vi "MegaAnalysis5.vi"() -> ()   [LabVIEW 2016] (continued)
                        tunnel: w4729 -> [w4829 w4834 w4839 w4845]
                        frame 0, Default {
                          n1882 = call "readbinary.vi"(7:w4829, "base path"=w4831, "file index"=w4832, "data column"="timi") -> ("data"=w4830:ext[])  [unwired: 7 out]
                        }
                        frame 1 {
                          n1883 = call "readbinary.vi"(7:w4834, "base path"=w4836, "file index"=w4837, "data column"="bcli") -> ("data"=w4835:ext[])  [unwired: 7 out]
                        }
                        frame 2 {
                          n1884 = call "readbinary.vi"(7:w4839, "base path"=w4842, "file index"=w4843, "data column"="bcli") -> ("data"=w4841:ext[])  [unwired: 7 out]
                          n1885 = Reciprocal(x=w4841) -> (1/x=w4840:ext[])
                        }
                        frame 3 {
                          n1886 = call "readbinary.vi"(7:w4845, "base path"=w4847, "file index"=w4848, "data column"="dati") -> ("data"=w4846:ext[])  [unwired: 7 out]
                        }
                      }
                      n1887 = case shown="2" w4736 {
                        tunnel: w4730 -> [w4811 w4816 w4822 w4827]
                        tunnel: w4732 -> [w4810 w4815 w4821 w4826]
                        tunnel: [w4809 w4814 w4819 w4825] -> w4727
                        tunnel: w4729 -> [w4808 w4813 w4818 w4824]
                        frame 0, Default {
                          n1888 = call "readbinary.vi"(7:w4808, "base path"=w4810, "file index"=w4811, "data column"="timi") -> ("data"=w4809:ext[])  [unwired: 7 out]
                        }
                        frame 1 {
                          n1889 = call "readbinary.vi"(7:w4813, "base path"=w4815, "file index"=w4816, "data column"="bcli") -> ("data"=w4814:ext[])  [unwired: 7 out]
                        }
                        frame 2 {
                          n1890 = call "readbinary.vi"(7:w4818, "base path"=w4821, "file index"=w4822, "data column"="bcli") -> ("data"=w4820:ext[])  [unwired: 7 out]
                          n1891 = Reciprocal(x=w4820) -> (1/x=w4819:ext[])
                        }
                        frame 3 {
                          n1892 = call "readbinary.vi"(7:w4824, "base path"=w4826, "file index"=w4827, "data column"="dati") -> ("data"=w4825:ext[])  [unwired: 7 out]
                        }
                      }
                      n1893 = Array Max & Min(array=w4727) -> (min value=w4726:ext)  [unwired: 3 out]
                      n1894 = case shown="0, Default" w4735 {
                        tunnel: w4734 -> [w4789 w4806]
                        tunnel: w4727 -> [w4786 w4807]
                        tunnel: w4733 -> [w4759 _]
                        tunnel: w4730 -> [w4770 w4802]
                        tunnel: w4732 -> [w4772 w4801]
                        tunnel: w4731 -> [w4768 _]
                        tunnel: w4728 -> [w4757 w4794]
                        tunnel: w4726 -> [w4749 _]
                        tunnel: w4725 -> [w4742 _]
                        frame 0, Default {
                          w4762 = 0
                          n1895 = Array Size(array=w4786) -> (size(s)=w4779:i32)
                          n1896 = Index Array(array=w4786, index=0) -> (element=w4784:ext)
                          n1897 = Decrement(x=w4779) -> (x-1=w4787:i32)
                          n1898 = Index Array(array=w4786, index=w4787) -> (element=w4783:ext)
                          n1899 = Subtract(x=w4784, y=w4783) -> (x-y=w4782:ext)
                          n1900 = Scale By Power Of 2(n=w4759, x=w4779) -> (x*2^n=w4766:i32)
                          n1901 = call-poly <vilib>:"Scaled Time Domain Window.vi"("window"="FT window", "X"=w4789) -> ("Windowed X"=w4750:dbl[])  [unwired: 1 in, 8 out]
                          n1902 = Scale By Power Of 2(n=w4759, x=1) -> (x*2^n=w4758:i32)
                          n1903 = Reciprocal(x=w4782) -> (1/x=w4780:ext)
                          n1904 = Subtract(x=w4766, y=w4779) -> (x-y=w4777:i32)
                          n1905 = Absolute Value(x=w4780) -> (abs(x)=w4781:ext)
                          n1906 = Array Size(array=w4750) -> (size(s)=w4755:i32)
                          n1907 = Divide(x=w4781, y=w4758) -> (x/y=w4775:ext)
                          n1908 = for {
                            N: w4777 -> [_]
                            tunnel: [0] -> w4778 mode=indexing
                          }
                          n1909 = Build Array (concatenate)(w4750, w4778) -> (w4756:dbl[])
                          n1910 = Divide(x=w4755, y=2) -> (x/y=w4753:dbl)
                          n1911 = call-poly <vilib>:"FFT.vi"("X"=w4756) -> ("FFT {X}"=w4752:cdb[])  [unwired: 2 in, 8 out]
                          n1912 = Divide(x=w4752, y=w4753) -> (x/y=w4751:cdb[])
                          n1913 = Complex To Polar(r * e^(i*theta)=w4751) -> (r=w4765:dbl[], theta=w4764:dbl[])
                          n1914 = for {
                            N: w4766 -> [w4790]
                            tunnel: [0] -> _ mode=indexing
                            tunnel: [w4791] -> w4776 mode=indexing
                            tunnel: [w4790] -> _ mode=indexing
                            i -> [w4791]
                          }
                          n1915 = Multiply(x=w4775, y=w4776) -> (x*y=w4763:ext[])
                          n1916 = Scale By Power Of 2(n=w4768, x=1) -> (x*2^n=w4767:i32)
                          n1917 = Divide(x=w4766, y=w4767) -> (x/y=w4761:dbl)
                          n1918 = Array Subset(array=w4765, index=w4762, length=w4761) -> (w4740:dbl[])
                          n1919 = Array Subset(array=w4764, index=w4762, length=w4761) -> (w4745:dbl[])
                          n1920 = Array Subset(array=w4763, index=w4762, length=w4761) -> (w4748:ext[])
                          n1921 = Multiply(x=w4748, y=w4749) -> (x*y=w4747:ext[])
                          n1922 = Multiply(x=w4747, y=6.283185307179586) -> (x*y=w4744:ext[])
                          n1923 = Multiply(x=w4744, y=w4742) -> (x*y=w4743:ext[])
                          n1924 = Subtract(x=w4745, y=w4743) -> (x-y=w4741:ext[])
                          n1925 = Polar To Complex(1:w4741, 2:w4740) -> (0:w4739:cxt[])
                          n1926 = call "writebinary.vi"(7:w4757, "base path"=w4772, "file index"=w4770, "data column"="freq", "data"=w4748) -> ()  [unwired: 7 out]
                          n1927 = Complex To Polar(r * e^(i*theta)=w4739) -> (theta=w4738:ext[])  [unwired: 1 out]
                          n1928 = call "writebinary.vi"(7:w4757, "base path"=w4772, "file index"=w4770, "data column"="ampl", "data"=w4740) -> ()  [unwired: 7 out]
                          n1929 = call "writebinary.vi"(7:w4757, "base path"=w4772, "file index"=w4770, "data column"="phas", "data"=w4738) -> ()  [unwired: 7 out]
                        }
                        frame 1 {
                          n1930 = call "MaxEnt03.vi"("t"=w4807, "data"=w4806, "m"="Maximum Entropy M", "pad factor?"="Increase spectral density") -> ("f"=w4800:dbl[], "P"=w4799:dbl[])  [unwired: 3 out]
                          n1931 = Square Root(x=w4799) -> (sqrt(x)=w4798:dbl[])
                          n1932 = call "writebinary.vi"(7:w4794, "base path"=w4801, "file index"=w4802, "data column"="freq", "data"=w4800) -> ()  [unwired: 7 out]
                          n1933 = call "writebinary.vi"(7:w4794, "base path"=w4801, "file index"=w4802, "data column"="ampl", "data"=w4798) -> ()  [unwired: 7 out]
                          n1934 = call "writebinary.vi"(7:w4794, "base path"=w4801, "file index"=w4802, "data column"="phas", "data"=dbl[] [] ("Array 16")) -> ()  [unwired: 7 out]
                        }
                      }
                    }
                  }
                  frame #2 {
                    n1935 = case shown="True" "?" {
                      tunnel: "peak finder threshold" -> [_ w4859]
                      tunnel: "width" -> [_ w4858]
                      tunnel: w4852 -> [_ w4861]
                      tunnel: w4851 -> [_ w4860]
                      tunnel: w4850 -> [_ w4856]
                      frame False {
                      }
                      frame True {
                        n1936 = for {
                          tunnel: w4861 -> [_] mode=indexing
                          tunnel: w4860 -> [w4878]
                          tunnel: w4859 -> [w4880]
                          tunnel: w4858 -> [w4871]
                          tunnel: [w4866] -> w4857 mode=indexing
                          tunnel: w4856 -> [w4862]
                          i -> [w4879]
                          (unwired) 0
                          n1937 = call "readbinary.vi"(7:w4862, "base path"=w4878, "file index"=w4879, "data column"="freq") -> ("data"=w4870:ext[])  [unwired: 7 out]
                          n1938 = call "readbinary.vi"(7:w4862, "base path"=w4878, "file index"=w4879, "data column"="ampl") -> ("data"=w4881:ext[])  [unwired: 7 out]
                          n1939 = call "readbinary.vi"(7:w4862, "base path"=w4878, "file index"=w4879, "data column"="phas") -> ("data"=w4869:ext[])  [unwired: 7 out]
                          n1940 = Index Array(array=w4870) -> (element=w4873:ext)  [unwired: 1 in]
                          n1941 = Index Array(array=w4870, index=1) -> (element=w4874:ext)
                          n1942 = Subtract(x=w4874, y=w4873) -> (x-y=w4872:ext)
                          n1943 = Divide(x=w4872, y=w4871) -> (x/y=w4868:ext)
                          n1944 = call-poly <vilib>:"Waveform Peak Detection.vi"("width"=w4868, "threshold"=w4880, "Signal In"=w4881) -> ("Amplitudes"=w4864:dbl[], "Locations"=w4867:dbl[])  [unwired: 4 in, 3 out]
                          n1945 = for {
                            tunnel: w4870 -> [w4888]
                            tunnel: w4869 -> [w4887]
                            tunnel: w4867 -> [w4886] mode=indexing
                            tunnel: w4867 -> [w4885] mode=indexing
                            tunnel: [w4884] -> w4865 mode=indexing
                            tunnel: [w4883] -> w4863 mode=indexing
                            n1946 = Index Array(array=w4888, index=w4885) -> (element=w4884:ext)
                            n1947 = Index Array(array=w4887, index=w4886) -> (element=w4883:ext)
                          }
                          n1948 = Bundle(w4863, w4865, "Amplitudes"=w4864) -> (w4866:cluster{ext[], ext[], "Amplitudes":dbl[]})  [unwired: 1 out]
                        }
                        "peaks" <- w4857
                      }
                    }
                  }
                }
              }
            }
          }
          frame #2 {
            n1949 = Equal?(x=w4899, y=4) -> (x = y?=w4896:bool)
            n1950 = Equal?(x="?", y=1) -> (x = y?=w4897:bool)
            n1951 = Build Path(base path=w4891, name or relative path="files4") -> (appended path=w4893:path)
            n1952 = call-poly <vilib>:"Read From Spreadsheet File.vi"("file path (dialog if empty)"=w4893) -> ("first row"=w4892:string[])  [unwired: 3 in, 7 out]
            n1953 = And(x=w4897, y=w4896) -> (x .and. y?=w4902:bool)
            n1954 = case shown="True" w4902 {
              tunnel: "y axis" -> [_ w4912]
              tunnel: w4892 -> [_ w4914]
              tunnel: w4891 -> [_ w4913]
              tunnel: [w4906 w4911] -> w4890
              tunnel: w4889 -> [_ w4910]
              frame False {
                w4908 = dbl[] [] ("Array 15")
                n1955 = Bundle("Array 15"=w4908, "Array 15"=w4908) -> (w4907:cluster{"Array 15":dbl[], "Array 15":dbl[]})  [unwired: 1 out]
                n1956 = Build Array(w4907) -> (w4906:cluster{"Array 15":dbl[], "Array 15":dbl[]}[])
              }
              frame True {
                n1957 = for {
                  tunnel: w4914 -> [_] mode=indexing
                  tunnel: w4913 -> [w4919]
                  tunnel: w4912 -> [w4921]
                  tunnel: [w4916] -> w4911 mode=indexing
                  tunnel: w4910 -> [w4915]
                  i -> [w4920]
                  n1958 = call "readbinary.vi"(7:w4915, "base path"=w4919, "file index"=w4920, "data column"="freq") -> ("data"=w4918:ext[])  [unwired: 7 out]
                  n1959 = case shown="2" w4921 {
                    tunnel: w4920 -> [w4926 w4932 w4937]
                    tunnel: w4919 -> [w4925 w4931 w4936]
                    tunnel: [w4924 w4929 w4935] -> w4917
                    tunnel: w4915 -> [w4923 w4928 w4934]
                    frame 0, Default {
                      n1960 = call "readbinary.vi"(7:w4923, "base path"=w4925, "file index"=w4926, "data column"="ampl") -> ("data"=w4924:ext[])  [unwired: 7 out]
                    }
                    frame 1 {
                      n1961 = call "readbinary.vi"(7:w4928, "base path"=w4931, "file index"=w4932, "data column"="ampl") -> ("data"=w4930:ext[])  [unwired: 7 out]
                      n1962 = Multiply(x=w4930, y=w4930) -> (x*y=w4929:ext[])
                    }
                    frame 2 {
                      n1963 = call "readbinary.vi"(7:w4934, "base path"=w4936, "file index"=w4937, "data column"="phas") -> ("data"=w4935:ext[])  [unwired: 7 out]
                    }
                  }
                  n1964 = Bundle("data"=w4918, "data"=w4917) -> (w4916:cluster{"data":ext[], "data":ext[]})  [unwired: 1 out]
                }
                n1965 = global write "status.vi" "String"("plotting transform") -> ()
              }
            }
            "?" <- w4890
            n1966 = while {
              stop <- w4904 stop-if-true
              n1967 = Not(x="?") -> (.not. x?=w4904:bool)
              n1968 = Wait (ms)(milliseconds to wait=1000) -> ()  [unwired: 1 out]
            }
          }
          frame #3 {
            w4941 = FALSE  # Set axes names
            n1969 = Build Path(base path=w4948, name or relative path="files4") -> (appended path=w4955:path)
            n1970 = Build Path(base path=w4948, name or relative path="paths4") -> (appended path=w4953:path)
            n1971 = call-poly <vilib>:"Read From Spreadsheet File.vi"("file path (dialog if empty)"=w4953) -> ("first row"=w4952:string[])  [unwired: 3 in, 7 out]
            n1972 = Build Array("freq", "ampl", "phas") -> (w4950:string[])
            n1973 = call-poly <vilib>:"Read From Spreadsheet File.vi"("file path (dialog if empty)"=w4955) -> ("first row"=w4944:string[])  [unwired: 3 in, 7 out]
            "files 2" <- w4944
            n1974 = case shown="0, Default" "label" {
              tunnel: w4944 -> [w4962 _ _]
              tunnel: [w4962 w4965 w4970] -> w4939
              frame 0, Default {
              }
              frame 1 {
                n1975 = property on="angle theta (cos theta renorm.)" class="Arr (strict)"() -> ("Value"=w4966:ext[])  [unwired: 2 in, 2 out]
                n1976 = Number To Fractional String(number=w4966, width (-)=10, precision (6)=3) -> (F-format string=w4965:string[])  [unwired: 1 out]
              }
              frame 2 {
                n1977 = property on="variable (T)" class="Arr (strict)"() -> ("Value"=w4969:dbl[])  [unwired: 2 in, 2 out]
                n1978 = Number To Fractional String(number=w4969, width (-)=10, precision (6)=3) -> (F-format string=w4970:string[])  [unwired: 1 out]
              }
            }
            n1979 = String To Path(string=w4952) -> (path=w4951:path[])
            n1980 = case shown="True" "?" {
              tunnel: w4944 -> [_ w4981]
              tunnel: w4951 -> [_ w4980]
              tunnel: w4950 -> [_ w4979]
              tunnel: w4948 -> [_ w4973]
              tunnel: "file format" -> [_ w4978]
              tunnel: "append name" -> [_ w4977]
              tunnel: w4947 -> [_ w4976]
              tunnel: w4946 -> [w4971 w4975]
              tunnel: [w4971 w4974] -> w4945
              frame False {
              }
              frame True {
                n1981 = for {
                  tunnel: w4981 -> [w4998] mode=indexing
                  tunnel: w4980 -> [w4996] mode=indexing
                  tunnel: w4977 -> [w4997]
                  tunnel: w4979 -> [w4994]
                  tunnel: w4973 -> [w4992]
                  tunnel: w4978 -> [w4989]
                  tunnel: w4976 -> [w4988]
                  shift-right: [w4984] -> w4974
                  shift-left: w4975 -> [w4986]
                  tunnel: w4973 -> [w4982]
                  i -> [w4993]
                  n1982 = call "filecount.vi"("Path"=w4982) -> ("file count string"=w4983:string)  [unwired: 10 in]
                  n1983 = Concatenate Strings("mega", w4983, w4998, w4997) -> (w4995:string)
                  n1984 = Build Path(base path=w4996, name or relative path=w4995) -> (appended path=w4985:path)
                  n1985 = Build Array (concatenate)(w4985, w4986) -> (w4984:path[])
                  n1986 = for {
                    tunnel: w4994 -> [w5010] mode=indexing
                    tunnel: w4993 -> [w5013]
                    tunnel: w4992 -> [w5012]
                    tunnel: [w5011] -> w4990 mode=indexing
                    tunnel: w4988 -> [w5009]
                    n1987 = call "readbinary.vi"(7:w5009, "base path"=w5012, "file index"=w5013, "data column"=w5010) -> ("data"=w5011:ext[])  [unwired: 7 out]
                  }
                  n1988 = stacked-sequence {
                    tunnel: "frequency\tamplitude\tphase\n" -> [_ w5004 _]
                    tunnel: w4985 -> [w4999 w5003 w5007]
                    tunnel: w4990 -> [_ _ w5008]
                    tunnel: w4989 -> [_ _ w5006]
                    frame #0 {
                      n1989 = call <vilib>:"Check if File or Folder Exists.vi"("path"=w4999) -> ("file or folder exists?"=w5000:bool)  [unwired: 1 in, 9 out]
                      n1990 = case shown="True" w5000 {
                        selector: w5000 -> [_ w5002]
                        tunnel: w4999 -> [_ w5001]
                        frame False {
                        }
                        frame True {
                          n1991 = Delete(path (use dialog)=w5001, entire hierarchy (F)=w5002) -> ()  [unwired: 1 in, 5 out]
                        }
                      }
                    }
                    frame #1 {
                      n1992 = Write to Text File(file (use dialog)=w5003, text=w5004) -> ()  [unwired: 1 in, 4 out]
                    }
                    frame #2 {
                      w5005 = TRUE
                      n1993 = call "Write To Spreadsheet File2.vi"("transpose? (no:F)"=w5005, "format (%d)"=w5006, "append to file? (new file:F)"=w5005, "2D data"=w5008, "file path (dialog if empty)"=w5007) -> ()  [unwired: 3 in, 1 out]
                    }
                  }
                }
                n1994 = global write "status.vi" "String"("saving transform") -> ()
              }
            }
            n1995 = control-ref of="?"() -> (w4940:refnum<vi>)
            n1996 = call "Neilsetplot.vi"("Set axes names"=w4941, "max # rows (-1:all)"=-1, "Plot names"=w4939, "XYGraph Refnum"=w4940) -> ()  [unwired: 6 in, 2 out]
          }
        }
      }
      frame #8 {
        # "analysis frame"
        n1997 = Build Path(base path=w5014, name or relative path="files3") -> (appended path=w5026:path)
        n1998 = Build Path(base path=w5014, name or relative path="files4") -> (appended path=w5034:path)
        n1999 = Equal?(x="?", y=1) -> (x = y?=w5029:bool)
        n2000 = call-poly <vilib>:"Read From Spreadsheet File.vi"("file path (dialog if empty)"=w5026) -> ("first row"=w5024:string[])  [unwired: 3 in, 7 out]
        n2001 = Equal?(x=w5030, y=5) -> (x = y?=w5028:bool)
        n2002 = call-poly <vilib>:"Read From Spreadsheet File.vi"("file path (dialog if empty)"=w5034) -> ("first row"=w5017:string[])  [unwired: 3 in, 7 out]
        n2003 = for {
          tunnel: w5017 -> [_] mode=indexing
          tunnel: [w5038] -> w5020 mode=indexing
          i -> [w5038]
        }
        n2004 = Number To Decimal String(number=w5020, width (-)=3) -> (decimal integer string=w5018:string[])
        n2005 = And(x=w5029, y=w5028) -> (x .and. y?=w5027:bool)
        n2006 = Build Array(w5018, w5017) -> (w5016:string[][])
        n2007 = Transpose 2D Array(2D array=w5016) -> (transposed array=→"file list":string[][])
        n2008 = stacked-sequence {
          tunnel: "?" -> [_ w5046 _ _]
          tunnel: w5036 -> [_ w5045 _ _]
          tunnel: w5014 -> [_ w5044 w5188 w5257]
          tunnel: w5017 -> [_ w5043 _ _]
          tunnel: w5027 -> [_ _ w5189 _]
          tunnel: w5024 -> [_ w5042 _ _]
          tunnel: w5023 -> [_ w5041 _ _]
          tunnel: w5022 -> [_ _ _ w5254]
          tunnel: [_ _ _ w5253] -> w5021
          frame #0 {
            n2009 = case shown="True" "set B angle as the variable?" {
              frame False {
              }
              frame True {
                n2010 = property on="angle theta (cos theta renorm.)" class="Arr (strict)"() -> ("Value"=w5040:ext[])  [unwired: 2 in, 2 out]
                n2011 = property on="variable (T)" class="Arr (strict)"("Val(Sgnl)"=w5040) -> ()  [unwired: 2 in, 2 out]
              }
            }
          }
          frame #1 {
            n2012 = case shown="True" w5046 {
              tunnel: w5044 -> [w5047 w5068]
              tunnel: w5045 -> [_ w5067]
              tunnel: w5043 -> [_ w5066]
              tunnel: w5042 -> [_ w5065]
              tunnel: w5041 -> [_ w5064]
              frame False {
                n2013 = Build Path(base path=w5047, name or relative path="afits") -> (appended path=w5052:path)
                n2014 = call <vilib>:"Check if File or Folder Exists.vi"("path"=w5052) -> ("file or folder exists?"=w5053:bool)  [unwired: 1 in, 9 out]
                n2015 = Build Path(base path=w5047, name or relative path="table") -> (appended path=w5055:path)
                n2016 = case shown="False" w5053 {
                  tunnel: w5052 -> [w5060 _]
                  frame False {
                    n2017 = call-poly <vilib>:"Write To Spreadsheet File.vi"("1D data"=string[] [] ("Array 20"), "file path (dialog if empty)"=w5060) -> ()  [unwired: 4 in, 3 out]
                  }
                  frame True {
                  }
                }
                n2018 = call <vilib>:"Check if File or Folder Exists.vi"("path"=w5055) -> ("file or folder exists?"=w5056:bool)  [unwired: 1 in, 9 out]
                n2019 = case shown="False" w5056 {
                  tunnel: w5055 -> [w5062 _]
                  frame False {
                    n2020 = call-poly <vilib>:"Write To Spreadsheet File.vi"("1D data"=string[] [] ("Array 18"), "file path (dialog if empty)"=w5062) -> ()  [unwired: 4 in, 3 out]
                  }
                  frame True {
                  }
                }
                n2021 = Build Path(base path=w5047, name or relative path="tfits") -> (appended path=w5049:path)
                n2022 = call <vilib>:"Check if File or Folder Exists.vi"("path"=w5049) -> ("file or folder exists?"=w5050:bool)  [unwired: 1 in, 9 out]
                n2023 = case shown="False" w5050 {
                  tunnel: w5049 -> [w5058 _]
                  frame False {
                    n2024 = call-poly <vilib>:"Write To Spreadsheet File.vi"("1D data"=string[] [] ("Array 21"), "file path (dialog if empty)"=w5058) -> ()  [unwired: 4 in, 3 out]
                  }
                  frame True {
                  }
                }
              }
              frame True {
                n2025 = stacked-sequence {
                  seq-local: [w5083 _] -> [_ w5131]
                  seq-local: ["variable (T)" _] -> [_ w5130]
                  tunnel: w5068 -> [w5086 w5133]
                  tunnel: w5067 -> [w5093 _]
                  tunnel: w5066 -> [w5087 _]
                  tunnel: w5065 -> [_ w5134]
                  tunnel: w5064 -> [_ w5132]
                  frame #0 {
                    w5072 = FALSE  # Set axes names
                    (unwired) 3
                    n2026 = for {
                      tunnel: w5087 -> [_] mode=indexing
                      tunnel: w5093 -> [w5109]
                      tunnel: w5086 -> [w5107]
                      tunnel: "variable (T)" -> [w5113] mode=indexing
                      tunnel: "frequencies" -> [w5114]
                      tunnel: [w5112] -> w5090 mode=indexing
                      tunnel: [w5111] -> w5083 mode=indexing
                      tunnel: "amplitude" -> [w5106]
                      tunnel: "phase" -> [w5104]
                      i -> [w5108]
                      n2027 = call "readbinary.vi"(7:w5109, "base path"=w5107, "file index"=w5108, "data column"="ampl") -> ("data"=w5102:ext[])  [unwired: 7 out]
                      n2028 = call "readbinary.vi"(7:w5109, "base path"=w5107, "file index"=w5108, "data column"="freq") -> ("data"=w5116:ext[])  [unwired: 7 out]
                      n2029 = call "readbinary.vi"(7:w5109, "base path"=w5107, "file index"=w5108, "data column"="phas") -> ("data"=w5103:ext[])  [unwired: 7 out]
                      n2030 = case shown="0, Default" w5106 {
                        tunnel: [w5119 w5120 w5125] -> w5105
                        tunnel: w5104 -> [_ w5123 w5128]
                        tunnel: w5103 -> [_ w5124 w5129]
                        tunnel: w5102 -> [w5119 w5122 w5127]
                        frame 0, Default {
                        }
                        frame 1 {
                          n2031 = Add(x=w5124, y=w5123) -> (x+y=w5121:ext[])
                          n2032 = Polar To Re/Im(2:w5121, 3:w5122) -> (1:w5120:ext[])  [unwired: 1 out]
                        }
                        frame 2 {
                          n2033 = Add(x=w5129, y=w5128) -> (x+y=w5126:ext[])
                          n2034 = Polar To Re/Im(2:w5126, 3:w5127) -> (0:w5125:ext[])  [unwired: 1 out]
                        }
                      }
                      n2035 = call <vilib>:"Interpolate 1D.vi"("method"="interpolation method", "xi"=w5114, "X"=w5116, "Y"=w5105) -> ("yi"=w5111:dbl[])  [unwired: 2 in, 5 out]
                      n2036 = Build Array (concatenate)(w5113, w5111) -> (w5112:dbl[])
                    }
                    n2037 = Build Array (concatenate)(0, "frequencies") -> (w5091:dbl[])
                    n2038 = control-ref of="?"() -> (w5070:refnum<vi>)
                    n2039 = Number To Fractional String(number="frequencies", width (-)=10, precision (6)=3) -> (F-format string=w5078:string[])  [unwired: 1 out]
                    n2040 = Build Array (concatenate)(w5091, w5090) -> (w5089:dbl[][])
                    n2041 = for {
                      tunnel: w5078 -> [w5101] mode=indexing
                      tunnel: [w5098] -> w5077 mode=indexing
                      tunnel: [w5097] -> w5076 mode=indexing
                      n2042 = Concatenate Strings("data ", w5101) -> (w5098:string)
                      n2043 = Concatenate Strings("fit ", w5101) -> (w5097:string)
                    }
                    n2044 = Build Path(base path=w5086, name or relative path="table") -> (appended path=w5084:path)
                    n2045 = call-poly <vilib>:"Write To Spreadsheet File.vi"("format (%.3f)"="%.9f", "2D data"=w5089, "file path (dialog if empty)"=w5084) -> ()  [unwired: 3 in, 3 out]
                    n2046 = Interleave 1D Arrays(w5077, w5076) -> (w5069:string[])
                    n2047 = call "Neilsetplot.vi"("Set axes names"=w5072, "max # rows (-1:all)"=20, "Plot names"=w5069, "XYGraph Refnum"=w5070) -> ()  [unwired: 6 in, 2 out]
                    n2048 = for {
                      tunnel: w5069 -> [w5096] mode=indexing
                      tunnel: [w5095] -> w5075 mode=indexing
                      n2049 = Bundle(w5096) -> (w5095:cluster{string})  [unwired: 1 in]
                    }
                    "frequencies" <- w5075
                    n2050 = for {
                      tunnel: [w5094] -> _ mode=indexing
                      tunnel: w5069 -> [_] mode=indexing
                      i -> [w5094]
                    }
                  }
                  frame #1 {
                    n2051 = case shown="False" "?" {
                      tunnel: w5134 -> [_ w5165]
                      tunnel: w5133 -> [w5136 w5149]
                      tunnel: w5132 -> [_ w5164]
                      tunnel: w5131 -> [_ w5162]
                      tunnel: w5130 -> [_ w5160]
                      frame False {
                        n2052 = Build Path(base path=w5136, name or relative path="afits") -> (appended path=w5141:path)
                        n2053 = call <vilib>:"Check if File or Folder Exists.vi"("path"=w5141) -> ("file or folder exists?"=w5142:bool)  [unwired: 1 in, 9 out]
                        n2054 = case shown="False" w5142 {
                          tunnel: w5141 -> [w5146 _]
                          frame False {
                            n2055 = call-poly <vilib>:"Write To Spreadsheet File.vi"("1D data"=string[] [] ("Array 22"), "file path (dialog if empty)"=w5146) -> ()  [unwired: 4 in, 3 out]
                          }
                          frame True {
                          }
                        }
                        n2056 = Build Path(base path=w5136, name or relative path="tfits") -> (appended path=w5138:path)
                        n2057 = call <vilib>:"Check if File or Folder Exists.vi"("path"=w5138) -> ("file or folder exists?"=w5139:bool)  [unwired: 1 in, 9 out]
                        n2058 = case shown="False" w5139 {
                          tunnel: w5138 -> [w5144 _]
                          frame False {
                            n2059 = call-poly <vilib>:"Write To Spreadsheet File.vi"("1D data"=string[] [] ("Array 23"), "file path (dialog if empty)"=w5144) -> ()  [unwired: 4 in, 3 out]
                          }
                          frame True {
                          }
                        }
                      }
                      frame True {
                        n2060 = for {
                          tunnel: w5165 -> [_] mode=indexing
                          tunnel: w5149 -> [w5184]
                          tunnel: w5164 -> [w5183]
                          tunnel: [w5173] -> w5163 mode=indexing
                          i -> [w5185]
                          n2061 = call "readbinary.vi"(7:w5183, "base path"=w5184, "file index"=w5185, "data column"="bcli") -> ("data"=w5181:ext[])  [unwired: 7 out]
                          n2062 = Array Max & Min(array=w5181) -> (max value=w5180:ext, min value=w5179:ext)  [unwired: 2 out]
                          n2063 = Reciprocal(x=w5179) -> (1/x=w5177:ext)
                          n2064 = Reciprocal(x=w5180) -> (1/x=w5178:ext)
                          n2065 = Add(x=w5178, y=w5177) -> (x+y=w5176:ext)
                          n2066 = Divide(x=w5176, y=2) -> (x/y=w5174:ext)
                          n2067 = Reciprocal(x=w5174) -> (1/x=w5173:ext)
                        }
                        n2068 = Transpose 2D Array(2D array=w5162) -> (transposed array=w5161:dbl[][])
                        n2069 = call-poly <vilib>:"Mean.vi"("X"=w5163) -> ("mean"=w5159:dbl)  [unwired: 1 out]
                        n2070 = for {
                          tunnel: w5161 -> [w5171] mode=indexing
                          tunnel: w5160 -> [w5172]
                          tunnel: w5159 -> [w5170]
                          tunnel: "points" -> [w5169]
                          tunnel: [w5168] -> w5157 mode=indexing
                          tunnel: [w5167] -> w5153 mode=indexing
                          tunnel: [w5166] -> w5148 mode=indexing
                          n2071 = call "sinh.vi"("# points"=w5169, "B"=w5170, "Amp"=w5171, "T"=w5172) -> ("mass"=w5168:dbl, "Amp"=w5166:dbl[], "T"=w5167:dbl[])  [unwired: 5 out]
                        }
                        n2072 = Absolute Value(x=w5157) -> (abs(x)=→"mass":dbl[])
                        n2073 = Build Path(base path=w5149, name or relative path="tfits") -> (appended path=w5154:path)
                        n2074 = call-poly <vilib>:"Write To Spreadsheet File.vi"("format (%.3f)"="%.9f", "2D data"=w5153, "file path (dialog if empty)"=w5154) -> ()  [unwired: 3 in, 3 out]
                        n2075 = Build Path(base path=w5149, name or relative path="afits") -> (appended path=w5150:path)
                        n2076 = call-poly <vilib>:"Write To Spreadsheet File.vi"("format (%.3f)"="%.9f", "2D data"=w5148, "file path (dialog if empty)"=w5150) -> ()  [unwired: 3 in, 3 out]
                      }
                    }
                  }
                }
                n2077 = global write "status.vi" "String"("amplitude analysis") -> ()
              }
            }
          }
          frame #2 {
            n2078 = case shown="False" w5189 {
              tunnel: w5188 -> [_ w5198]
              tunnel: [w5191 w5199] -> w5187
              tunnel: [0 3000] -> w5186
              frame False {
                w5193 = dbl[] [] ("Array 19")
                n2079 = Bundle("Array 19"=w5193, "Array 19"=w5193) -> (w5192:cluster{"Array 19":dbl[], "Array 19":dbl[]})  [unwired: 1 out]
                n2080 = Build Array(w5192) -> (w5191:cluster{"Array 19":dbl[], "Array 19":dbl[]}[])
              }
              frame True {
                w5222 = 1
                n2081 = Build Path(base path=w5198, name or relative path="tfits") -> (appended path=w5211:path)
                n2082 = Build Path(base path=w5198, name or relative path="afits") -> (appended path=w5208:path)
                n2083 = call-poly <vilib>:"Read From Spreadsheet File.vi"("format (%.3f)"="%.9f", "file path (dialog if empty)"=w5211) -> ("all rows"=w5205:dbl[][])  [unwired: 2 in, 7 out]
                n2084 = call-poly <vilib>:"Read From Spreadsheet File.vi"("format (%.3f)"="%.9f", "file path (dialog if empty)"=w5208) -> ("all rows"=w5204:dbl[][])  [unwired: 2 in, 7 out]
                n2085 = Build Path(base path=w5198, name or relative path="table") -> (appended path=w5227:path)
                n2086 = call-poly <vilib>:"Read From Spreadsheet File.vi"("format (%.3f)"="%.9f", "file path (dialog if empty)"=w5227) -> ("all rows"=w5218:dbl[][])  [unwired: 2 in, 7 out]
                n2087 = Index Array(array=w5218, index (col)=0) -> (element=w5216:dbl[])  [unwired: 1 in]
                n2088 = for {
                  tunnel: w5205 -> [w5249] mode=indexing
                  tunnel: w5204 -> [w5248] mode=indexing
                  tunnel: [w5247] -> w5197 mode=indexing
                  n2089 = Bundle("all rows"=w5249, "all rows"=w5248) -> (w5247:cluster{"all rows":dbl[], "all rows":dbl[]})  [unwired: 1 out]
                }
                n2090 = Array Size(array=w5218) -> (size(s)=w5224:i32[])
                n2091 = Index Array(array=w5224, index=1) -> (element=w5223:i32)
                n2092 = Index Array(array=w5224, index=0) -> (element=w5214:i32)
                n2093 = Array Subset(array=w5216, index=1, length=w5214) -> (w5213:dbl[])
                n2094 = global write "status.vi" "String"("plotting") -> ()
                n2095 = Decrement(x=w5214) -> ()  [unwired: 1 out]
                n2096 = Decrement(x=w5223) -> (x-1=w5221:i32)
                n2097 = Array Subset(array=w5218, index (row)=w5222, length (row)=w5214, index (col)=w5222, length (col)=w5221) -> (w5220:dbl[][])
                n2098 = Transpose 2D Array(2D array=w5220) -> (transposed array=w5219:dbl[][])
                n2099 = for {
                  tunnel: w5219 -> [w5251] mode=indexing
                  tunnel: w5213 -> [w5252]
                  tunnel: [w5250] -> w5196 mode=indexing
                  n2100 = Bundle(w5252, w5251) -> (w5250:cluster{dbl[], dbl[]})  [unwired: 1 out]
                }
                n2101 = Array Size(array=w5196) -> (size(s)=w5202:i32)
                n2102 = Multiply(x=2, y=w5202) -> (x*y=w5200:i32)
                n2103 = for {
                  N: w5200 -> [_]
                  tunnel: w5197 -> [w5232]
                  tunnel: w5196 -> [w5233]
                  shift-right: [w5235] -> _
                  shift-left: 0 -> [w5230]
                  tunnel: [w5231] -> w5199 mode=indexing
                  i -> [w5229]
                  n2104 = case shown="0, Default" w5230 {
                    tunnel: w5229 -> [w5239 w5246]
                    tunnel: w5233 -> [w5238 _]
                    tunnel: [w5236 w5242] -> w5231
                    tunnel: w5232 -> [_ w5243]
                    frame 0, Default {
                      n2105 = Divide(x=w5239, y=2) -> (x/y=w5237:dbl)
                      n2106 = Index Array(array=w5238, index=w5237) -> (element=w5236:cluster{dbl[], dbl[]})
                    }
                    frame 1 {
                      n2107 = Decrement(x=w5246) -> (x-1=w5245:i32)
                      n2108 = Divide(x=w5245, y=2) -> (x/y=w5244:dbl)
                      n2109 = Index Array(array=w5243, index=w5244) -> (element=w5242:cluster{"all rows":dbl[], "all rows":dbl[]})
                    }
                  }
                  n2110 = Subtract(x=1, y=w5230) -> (x-y=w5235:i32)
                }
              }
            }
            "?" <- w5187
            n2111 = Wait (ms)(milliseconds to wait=w5186) -> ()  [unwired: 1 out]
          }
          frame #3 {
            n2112 = Build Path(base path=w5257, name or relative path="paths4") -> (appended path=w5258:path)
            n2113 = call-poly <vilib>:"Read From Spreadsheet File.vi"("file path (dialog if empty)"=w5258) -> ("first row"=w5256:string[])  [unwired: 3 in, 7 out]
            n2114 = String To Path(string=w5256) -> (path=w5255:path[])
            n2115 = case shown="True" "?" {
              tunnel: w5257 -> [_ w5273]
              tunnel: w5255 -> [_ w5275]
              tunnel: w5254 -> [w5261 w5265]
              tunnel: [w5261 w5263] -> w5253
              frame False {
              }
              frame True {
                n2116 = Index Array(array=w5275, index=0) -> (element=w5268:path)
                n2117 = call "filecount.vi"("Path"=w5273) -> ("file count string"=w5271:string)  [unwired: 10 out]
                n2118 = Build Path(base path=w5273, name or relative path="table") -> (appended path=w5277:path)
                n2119 = call-poly <vilib>:"Read From Spreadsheet File.vi"("format (%.3f)"="%.9f", "file path (dialog if empty)"=w5277) -> ("all rows"=w5267:dbl[][])  [unwired: 2 in, 7 out]
                n2120 = Concatenate Strings("mega", w5271, "append name") -> (w5269:string)
                n2121 = Build Path(base path=w5268, name or relative path=w5269) -> (appended path=w5264:path)
                n2122 = Build Array (concatenate)(w5264, w5265) -> (w5263:path[])
                n2123 = call "Write To Spreadsheet File2.vi"("format (%d)"="file format", "2D data"=w5267, "file path (dialog if empty)"=w5264) -> ()  [unwired: 5 in, 1 out]
                n2124 = global write "status.vi" "String"("saving analysis") -> ()
              }
            }
          }
        }
      }
      frame #9 {
        n2125 = stacked-sequence {
          seq-local: [w5280 _ _ _ _ _ _ _] -> [_ _ _ _ _ _ w5529 _]
          seq-local: [_ w5287 _ _ _ _ _ _] -> [_ _ _ _ _ _ w5528 _]
          seq-local: [_ _ w5380 _ _ _ _ _] -> [_ _ _ _ _ _ w5527 _]
          seq-local: [_ _ _ w5434 _ _ _ _] -> [_ _ _ _ _ _ w5526 _]
          seq-local: [_ _ _ _ w5486 _ _ _] -> [_ _ _ _ _ _ w5525 _]
          seq-local: [_ _ _ _ _ w5505 _ _] -> [_ _ _ _ _ _ w5524 _]
          seq-local: [_ _ _ _ _ _ w5522 _] -> [_ _ _ _ _ _ _ w5533]
          seq-local: [_ _ _ _ _ _ w5519 _] -> [_ _ _ _ _ _ _ w5532]
          tunnel: "?" -> [_ _ _ _ _ _ _ w5534]
          frame #0 {
            # "transform"
            # "interpolate"
            # "select"
            # "filter"
            # "import"
            # "pruge"
            n2126 = property class="Bool (strict)"() -> ("Value"=w5286:bool)  [unwired: 2 in, 2 out]
            n2127 = property class="Bool (strict)"() -> ("Value"=w5285:bool)  [unwired: 2 in, 2 out]
            n2128 = property class="Bool (strict)"() -> ("Value"=w5283:bool)  [unwired: 2 in, 2 out]
            n2129 = property class="Bool (strict)"() -> ("Value"=w5284:bool)  [unwired: 2 in, 2 out]
            n2130 = property class="Bool (strict)"() -> ("Value"=w5281:bool)  [unwired: 2 in, 2 out]
            n2131 = property class="Bool (strict)"() -> ("Value"=w5282:bool)  [unwired: 2 in, 2 out]
            n2132 = Bundle("Value"=w5286, "Value"=w5285, "Value"=w5284, "Value"=w5283, "Value"=w5282, "Value"=w5281) -> (w5280:T19)  [unwired: 1 out]
          }
          frame #1 {
            n2133 = stacked-sequence {
              seq-local: [w5292 _ _ _ _ _] -> [_ _ _ _ _ w5379]
              seq-local: [_ w5293 _ _ _ _] -> [_ _ _ _ _ w5378]
              seq-local: [_ _ w5345 _ _ _] -> [_ _ _ _ _ w5377]
              seq-local: [_ _ _ w5356 _ _] -> [_ _ _ _ _ w5376]
              seq-local: [_ _ _ _ w5371 _] -> [_ _ _ _ _ w5375]
              tunnel: [_ _ _ _ _ w5374] -> w5291
              frame #0 {
                n2134 = property on="files to be imported" class="Arr (strict)"() -> ("Value"=w5292:path[])  [unwired: 2 in, 2 out]
              }
              frame #1 {
                # "integration pretrigger option"
                n2135 = stacked-sequence {
                  tunnel: [w5301 _ _ _ _] -> w5298
                  tunnel: [_ w5307 _ _ _] -> w5297
                  tunnel: [_ _ w5315 _ _] -> w5296
                  tunnel: [_ _ _ w5324 _] -> w5295
                  tunnel: [_ _ _ _ w5334] -> w5294
                  frame #0 {
                    n2136 = property on="time interval  (for series)" class="DigNum (strict)"() -> ("Value"=w5304:dbl)  [unwired: 2 in, 2 out]
                    n2137 = property on="time column selection" class="Arr (strict)"() -> ("Value"=w5303:u16[])  [unwired: 2 in, 2 out]
                    n2138 = property on="time column rescale" class="Arr (strict)"() -> ("Value"=w5302:ext[])  [unwired: 2 in, 2 out]
                    n2139 = property on="option" class="Ring (strict)"() -> ("Value"=w5305:u16)  [unwired: 2 in, 2 out]
                    n2140 = Bundle("Value"=w5305, "Value"=w5304, "Value"=w5303, "Value"=w5302) -> (w5301:T20)  [unwired: 1 out]
                  }
                  frame #1 {
                    n2141 = property on="dB/dt column rescale" class="Arr (strict)"() -> ("Value"=w5308:ext[])  [unwired: 2 in, 2 out]
                    n2142 = property on="dB/dt column selection" class="Arr (strict)"() -> ("Value"=w5309:u16[])  [unwired: 2 in, 2 out]
                    n2143 = property on="option" class="Ring (strict)"() -> ("Value"=w5310:u16)  [unwired: 2 in, 2 out]
                    n2144 = property class="Bool (strict)"() -> ("Value"=w5306:bool)  [unwired: 2 in, 2 out]
                    n2145 = Bundle("Value"=w5310, "Value"=w5309, "Value"=w5308, "Value"=w5306) -> (w5307:T21)  [unwired: 1 out]
                  }
                  frame #2 {
                    n2146 = local read "B column selection"() -> (w5311:u16[])
                    n2147 = property on="B column offset" class="Arr (strict)"() -> ("Value"=w5319:ext[])  [unwired: 2 in, 2 out]
                    n2148 = property on="angle theta (cos theta renorm.)" class="Arr (strict)"() -> ("Value"=w5320:ext[])  [unwired: 2 in, 2 out]
                    n2149 = property on="B column rescale" class="Arr (strict)"() -> ("Value"=w5321:ext[])  [unwired: 2 in, 2 out]
                    n2150 = property on="pretrigger time for integration" class="DigNum (strict)"() -> ("Value"=w5322:dbl)  [unwired: 2 in, 2 out]
                    n2151 = property on="option" class="Ring (strict)"() -> ("Value"=w5323:u16)  [unwired: 2 in, 2 out]
                    n2152 = property class="Bool (strict)"() -> ("Value"=w5317:bool)  [unwired: 2 in, 2 out]
                    n2153 = property class="Bool (strict)"() -> ("Value"=w5318:bool)  [unwired: 2 in, 2 out]
                    n2154 = property class="Bool (strict)"() -> ("Value"=w5316:bool)  [unwired: 2 in, 2 out]
                    n2155 = property class="Bool (strict)"() -> ("Value"=w5314:bool)  [unwired: 2 in, 2 out]
                    n2156 = property class="DigNum (strict)"() -> ("Value"=w5313:u32)  [unwired: 2 in, 2 out]
                    n2157 = property class="DigNum (strict)"() -> ("Value"=w5312:dbl)  [unwired: 2 in, 2 out]
                    n2158 = Bundle("Value"=w5323, "Value"=w5322, "B column selection"=w5311, "Value"=w5321, "Value"=w5320, "Value"=w5319, "Value"=w5318, "Value"=w5317, "Value"=w5316, "Value"=w5314, "Value"=w5313, "Value"=w5312) -> (w5315:T22)  [unwired: 1 out]
                  }
                  frame #3 {
                    # "rotate array"
                    n2159 = property on="pretrigger time for integration" class="DigNum (strict)"() -> ("Value"=w5332:dbl)  [unwired: 2 in, 2 out]
                    n2160 = property on="data column rescale" class="Arr (strict)"() -> ("Value"=w5328:ext[])  [unwired: 2 in, 2 out]
                    n2161 = property class="Bool (strict)"() -> ("Value"=w5331:bool)  [unwired: 2 in, 2 out]
                    n2162 = property on="data column selection" class="Arr (strict)"() -> ("Value"=w5329:u16[])  [unwired: 2 in, 2 out]
                    n2163 = property on="option" class="Ring (strict)"() -> ("Value"=w5333:u16)  [unwired: 2 in, 2 out]
                    n2164 = property class="DigNum (strict)"() -> ("Value"=w5330:i64)  [unwired: 2 in, 2 out]
                    n2165 = property on="data column offset" class="Arr (strict)"() -> ("Value"=w5327:ext[])  [unwired: 2 in, 2 out]
                    n2166 = property class="Bool (strict)"() -> ("Value"=w5326:bool)  [unwired: 2 in, 2 out]
                    n2167 = property class="Bool (strict)"() -> ("Value"=w5325:bool)  [unwired: 2 in, 2 out]
                    n2168 = Bundle("Value"=w5333, "Value"=w5332, "Value"=w5331, "Value"=w5330, "Value"=w5329, "Value"=w5328, "Value"=w5327, "Value"=w5326, "Value"=w5325) -> (w5324:T23)  [unwired: 1 out]
                  }
                  frame #4 {
                    n2169 = property on="pretrigger time for integration" class="DigNum (strict)"() -> ("Value"=w5342:dbl)  [unwired: 2 in, 2 out]
                    n2170 = property on="option" class="Ring (strict)"() -> ("Value"=w5343:u16)  [unwired: 2 in, 2 out]
                    n2171 = property class="Bool (strict)"() -> ("Value"=w5341:bool)  [unwired: 2 in, 2 out]
                    n2172 = property on="data column rescale" class="Arr (strict)"() -> ("Value"=w5338:ext[])  [unwired: 2 in, 2 out]
                    n2173 = property class="DigNum (strict)"() -> ("Value"=w5340:i64)  [unwired: 2 in, 2 out]
                    n2174 = property on="data column selection" class="Arr (strict)"() -> ("Value"=w5339:u16[])  [unwired: 2 in, 2 out]
                    n2175 = property on="data column offset" class="Arr (strict)"() -> ("Value"=w5337:ext[])  [unwired: 2 in, 2 out]
                    n2176 = property class="Bool (strict)"() -> ("Value"=w5336:bool)  [unwired: 2 in, 2 out]
                    n2177 = property class="Bool (strict)"() -> ("Value"=w5335:bool)  [unwired: 2 in, 2 out]
                    n2178 = Bundle("Value"=w5343, "Value"=w5342, "Value"=w5341, "Value"=w5340, "Value"=w5339, "Value"=w5338, "Value"=w5337, "Value"=w5336, "Value"=w5335) -> (w5334:T23)  [unwired: 1 out]
                  }
                }
                n2179 = property on="column selection options (for each file)" class="Ring (strict)"() -> ("Value"=w5300:u16)  [unwired: 2 in, 2 out]
                n2180 = property class="Bool (strict)"() -> ("Value"=w5299:bool)  [unwired: 2 in, 2 out]
                n2181 = Bundle("Value"=w5300, "Value"=w5299, w5298, w5297, w5296, w5295, w5294) -> (w5293:T24)  [unwired: 1 out]
              }
              frame #2 {
                n2182 = property class="Bool (strict)"() -> ("Value"=w5353:bool)  [unwired: 2 in, 2 out]
                n2183 = property class="Bool (strict)"() -> ("Value"=w5354:bool)  [unwired: 2 in, 2 out]
                n2184 = property class="Bool (strict)"() -> ("Value"=w5352:bool)  [unwired: 2 in, 2 out]
                n2185 = property on="lower cutoff" class="DigNum (strict)"() -> ("Value"=w5350:ext)  [unwired: 2 in, 2 out]
                n2186 = property on="lower cutoff" class="DigNum (strict)"() -> ("Value"=w5351:u64)  [unwired: 2 in, 2 out]
                n2187 = property on="lower cutoff" class="DigNum (strict)"() -> ("Value"=w5349:ext)  [unwired: 2 in, 2 out]
                n2188 = property on="upper cutoff" class="DigNum (strict)"() -> ("Value"=w5348:u64)  [unwired: 2 in, 2 out]
                n2189 = property on="upper cutoff" class="DigNum (strict)"() -> ("Value"=w5347:ext)  [unwired: 2 in, 2 out]
                n2190 = property on="upper cutoff" class="DigNum (strict)"() -> ("Value"=w5346:ext)  [unwired: 2 in, 2 out]
                n2191 = property class="Bool (strict)"() -> ("Value"=w5344:bool)  [unwired: 2 in, 2 out]
                n2192 = Bundle("Value"=w5354, "Value"=w5353, "Value"=w5352, "Value"=w5351, "Value"=w5350, "Value"=w5349, "Value"=w5348, "Value"=w5347, "Value"=w5346, "Value"=w5344) -> (w5345:T25)  [unwired: 1 out]
              }
              frame #3 {
                n2193 = property on="filter selection" class="Ring (strict)"() -> ("Value"=w5370:u16)  [unwired: 2 in, 2 out]
                n2194 = property on="sampling frequency option" class="Ring (strict)"() -> ("Value"=w5369:u16)  [unwired: 2 in, 2 out]
                n2195 = property on="sampling frequency" class="Arr (strict)"() -> ("Value"=w5368:dbl[])  [unwired: 2 in, 2 out]
                n2196 = property on="window" class="Ring (strict)"() -> ("Value"=w5360:i32)  [unwired: 2 in, 2 out]
                n2197 = property on="attenuation (dB)" class="DigNum (strict)"() -> ("Value"=w5362:dbl)  [unwired: 2 in, 2 out]
                n2198 = property on="passband ripple (dB)" class="DigNum (strict)"() -> ("Value"=w5361:dbl)  [unwired: 2 in, 2 out]
                n2199 = property on="filter type" class="Enum (strict)"() -> ("Value"=w5367:T5)  [unwired: 2 in, 2 out]
                n2200 = property on="order" class="DigNum (strict)"() -> ("Value"=w5364:i32)  [unwired: 2 in, 2 out]
                n2201 = property on="ripple(dB)" class="DigNum (strict)"() -> ("Value"=w5363:dbl)  [unwired: 2 in, 2 out]
                n2202 = property on="left rank" class="DigNum (strict)"() -> ("Value"=w5358:i32)  [unwired: 2 in, 2 out]
                n2203 = property on="low cutoff freq: fl" class="DigNum (strict)"() -> ("Value"=w5366:dbl)  [unwired: 2 in, 2 out]
                n2204 = property on="taps" class="DigNum (strict)"() -> ("Value"=w5359:i32)  [unwired: 2 in, 2 out]
                n2205 = property on="right rank" class="DigNum (strict)"() -> ("Value"=w5357:i32)  [unwired: 2 in, 2 out]
                n2206 = property on="stopband attenuation (dB)" class="DigNum (strict)"() -> ("Value"=w5355:dbl)  [unwired: 2 in, 2 out]
                n2207 = property on="high cutoff freq: fh" class="DigNum (strict)"() -> ("Value"=w5365:dbl)  [unwired: 2 in, 2 out]
                n2208 = Bundle("Value"=w5370, "Value"=w5369, "Value"=w5368, "Value"=w5367, "Value"=w5366, "Value"=w5365, "Value"=w5364, "Value"=w5363, "Value"=w5362, "Value"=w5361, "Value"=w5360, "Value"=w5359, "Value"=w5358, "Value"=w5357, "Value"=w5355) -> (w5356:T26)  [unwired: 1 out]
              }
              frame #4 {
                n2209 = property on="append name" class="Str"() -> ("Value"=w5373:string)  [unwired: 2 in, 2 out]
                n2210 = property class="Bool (strict)"() -> ("Value"=w5372:bool)  [unwired: 2 in, 2 out]
                n2211 = Bundle("Value"=w5373, "Value"=w5372) -> (w5371:cluster{"Value":string, "Value":bool})  [unwired: 1 out]
              }
              frame #5 {
                n2212 = Bundle("Value"=w5379, w5378, w5377, w5376, w5375) -> (w5374:T27)  [unwired: 1 out]
              }
            }
            n2213 = property on="skip" class="DigNum (strict)"() -> ("Value"=w5289:u16)  [unwired: 2 in, 2 out]
            n2214 = property class="Ring (strict)"() -> ("Value"=w5290:u16)  [unwired: 2 in, 2 out]
            n2215 = property on="file format" class="Str"() -> ("Value"=w5288:string)  [unwired: 2 in, 2 out]
            n2216 = Bundle("Value"=w5290, "Value"=w5289, "Value"=w5288, w5291) -> (w5287:T28)  [unwired: 1 out]
          }
          frame #2 {
            n2217 = stacked-sequence {
              seq-local: [w5383 _ _ _ _ _ _] -> [_ _ _ _ _ _ w5433]
              seq-local: [_ w5388 _ _ _ _ _] -> [_ _ _ _ _ _ w5432]
              seq-local: [_ _ w5393 _ _ _ _] -> [_ _ _ _ _ _ w5431]
              seq-local: [_ _ _ w5408 _ _ _] -> [_ _ _ _ _ _ w5430]
              seq-local: [_ _ _ _ _ w5426 _] -> [_ _ _ _ _ _ w5429]
              seq-local: [_ _ _ _ w5420 _ _] -> [_ _ _ _ _ _ w5427]
              tunnel: [_ _ _ _ _ _ w5428] -> w5381
              frame #0 {
                n2218 = property class="Bool (strict)"() -> ("Value"=w5387:bool)  [unwired: 2 in, 2 out]
                n2219 = property on="reference option" class="Ring (strict)"() -> ("Value"=w5386:u16)  [unwired: 2 in, 2 out]
                n2220 = property on="file name options" class="Ring (strict)"() -> ("Value"=w5385:u16)  [unwired: 2 in, 2 out]
                n2221 = property class="DigNum (strict)"() -> ("Value"=w5384:u8)  [unwired: 2 in, 2 out]
                n2222 = Bundle("Value"=w5387, "Value"=w5386, "Value"=w5385, "Value"=w5384) -> (w5383:T29)  [unwired: 1 out]
              }
              frame #1 {
                n2223 = property class="Bool (strict)"() -> ("Value"=w5392:bool)  [unwired: 2 in, 2 out]
                n2224 = property class="Bool (strict)"() -> ("Value"=w5390:bool)  [unwired: 2 in, 2 out]
                n2225 = property on="append string onto file name" class="Str"() -> ("Value"=w5391:string)  [unwired: 2 in, 2 out]
                n2226 = property class="DigNum (strict)"() -> ("Value"=w5389:u8)  [unwired: 2 in, 2 out]
                n2227 = Bundle("Value"=w5392, "Value"=w5391, "Value"=w5390, "Value"=w5389) -> (w5388:T30)  [unwired: 1 out]
              }
              frame #2 {
                n2228 = property on="data options" class="Ring (strict)"() -> ("Value"=w5404:u16)  [unwired: 2 in, 2 out]
                n2229 = property class="Bool (strict)"() -> ("Value"=w5403:bool)  [unwired: 2 in, 2 out]
                n2230 = property class="DigNum (strict)"() -> ("Value"=w5402:dbl)  [unwired: 2 in, 2 out]
                n2231 = property class="Bool (strict)"() -> ("Value"=w5399:bool)  [unwired: 2 in, 2 out]
                n2232 = property class="Bool (strict)"() -> ("Value"=w5395:bool)  [unwired: 2 in, 2 out]
                n2233 = property class="Bool (strict)"() -> ("Value"=w5401:bool)  [unwired: 2 in, 2 out]
                n2234 = property class="Bool (strict)"() -> ("Value"=w5397:bool)  [unwired: 2 in, 2 out]
                n2235 = property class="DigNum (strict)"() -> ("Value"=w5394:dbl)  [unwired: 2 in, 2 out]
                n2236 = property class="DigNum (strict)"() -> ("Value"=w5400:dbl)  [unwired: 2 in, 2 out]
                n2237 = property class="DigNum (strict)"() -> ("Value"=w5396:dbl)  [unwired: 2 in, 2 out]
                n2238 = property class="DigNum (strict)"() -> ("Value"=w5398:dbl)  [unwired: 2 in, 2 out]
                n2239 = Bundle("Value"=w5404, "Value"=w5403, "Value"=w5402, "Value"=w5401, "Value"=w5400, "Value"=w5399, "Value"=w5398, "Value"=w5397, "Value"=w5396, "Value"=w5395, "Value"=w5394) -> (w5393:T31)  [unwired: 1 out]
              }
              frame #3 {
                n2240 = property on="field limits:" class="Ring (strict)"() -> ("Value"=w5405:u16)  [unwired: 2 in, 2 out]
                n2241 = property class="Bool (strict)"() -> ("Value"=w5419:bool)  [unwired: 2 in, 2 out]
                n2242 = property on="threshold # of points below which field variations are ignored" class="DigNum (strict)"() -> ("Value"=w5415:dbl)  [unwired: 2 in, 2 out]
                n2243 = property on="row" class="Arr (strict)"() -> ("Value"=w5412:dbl[][])  [unwired: 2 in, 2 out]
                n2244 = property on="(slow on large data sets but good for treating small fluctuations in field)" class="DigNum (strict)"() -> ("Value"=w5418:dbl)  [unwired: 2 in, 2 out]
                n2245 = property class="Arr (strict)"() -> ("Value"=w5417:cluster{dbl, "and":dbl}[])  [unwired: 2 in, 2 out]
                n2246 = property on="fields" class="Arr (strict)"() -> ("Value"=w5411:dbl[][])  [unwired: 2 in, 2 out]
                n2247 = property on="maxima above:" class="DigNum (strict)"() -> ("Value"=w5407:dbl)  [unwired: 2 in, 2 out]
                n2248 = property on="consider variations in B field only above:" class="DigNum (strict)"() -> ("Value"=w5414:dbl)  [unwired: 2 in, 2 out]
                n2249 = property class="Bool (strict)"() -> ("Value"=w5416:bool)  [unwired: 2 in, 2 out]
                n2250 = property on="rising sweep start index" class="Arr (strict)"() -> ("Value"=w5410:dbl[])  [unwired: 2 in, 2 out]
                n2251 = property on="minima below :" class="DigNum (strict)"() -> ("Value"=w5406:dbl)  [unwired: 2 in, 2 out]
                n2252 = property class="Bool (strict)"() -> ("Value"=w5413:bool)  [unwired: 2 in, 2 out]
                n2253 = property on="falling sweep start index" class="Arr (strict)"() -> ("Value"=w5409:dbl[])  [unwired: 2 in, 2 out]
                n2254 = Bundle("Value"=w5419, "Value"=w5418, "Value"=w5405, "Value"=w5417, "Value"=w5416, "Value"=w5415, "Value"=w5414, "Value"=w5413, "Value"=w5412, "Value"=w5411, "Value"=w5410, "Value"=w5409, "Value"=w5407, "Value"=w5406) -> (w5408:T32)  [unwired: 1 out]
              }
              frame #4 {
                n2255 = property on="offset options" class="Ring (strict)"() -> ("Value"=w5423:u16)  [unwired: 2 in, 2 out]
                n2256 = property on="field smoothing" class="Ring (strict)"() -> ("Value"=w5425:u16)  [unwired: 2 in, 2 out]
                n2257 = property on="offset value" class="DigNum (strict)"() -> ("Value"=w5422:dbl)  [unwired: 2 in, 2 out]
                n2258 = property on="smoothing ratio (must be appreciably larger than 1)" class="DigNum (strict)"() -> ("Value"=w5424:u8)  [unwired: 2 in, 2 out]
                n2259 = property on="sweeprate-dependent  offset multiplier" class="DigNum (strict)"() -> ("Value"=w5421:dbl)  [unwired: 2 in, 2 out]
                n2260 = Bundle("Value"=w5425, "Value"=w5424, "Value"=w5423, "Value"=w5422, "Value"=w5421) -> (w5420:T33)  [unwired: 1 out]
              }
              frame #5 {
                n2261 = property on="append name" class="Str"() -> ("Value"=w5426:string)  [unwired: 2 in, 2 out]
              }
              frame #6 {
                n2262 = Bundle(w5433, w5432, w5431, w5430, "Value"=w5429, w5427) -> (w5428:T34)  [unwired: 1 out]
              }
            }
            n2263 = property class="Ring (strict)"() -> ("Value"=w5382:u16)  [unwired: 2 in, 2 out]
            n2264 = Bundle("Value"=w5382, w5381) -> (w5380:T35)  [unwired: 1 out]
          }
          frame #3 {
            n2265 = stacked-sequence {
              seq-local: [w5438 _ _ _ _ _] -> [_ _ _ _ _ w5485]
              seq-local: [_ w5447 _ _ _ _] -> [_ _ _ _ _ w5484]
              seq-local: [_ _ w5466 _ _ _] -> [_ _ _ _ _ w5483]
              seq-local: [_ _ _ w5470 _ _] -> [_ _ _ _ _ w5482]
              seq-local: [_ _ _ _ w5475 _] -> [_ _ _ _ _ w5481]
              tunnel: [_ _ _ _ _ w5480] -> w5435
              frame #0 {
                n2266 = property on="interpolate in:" class="Ring (strict)"() -> ("Value"=w5442:u16)  [unwired: 2 in, 2 out]
                n2267 = property on="rising and falling field options" class="Ring (strict)"() -> ("Value"=w5439:u16)  [unwired: 2 in, 2 out]
                n2268 = property on="# points" class="DigNum (strict)"() -> ("Value"=w5441:u64)  [unwired: 2 in, 2 out]
                n2269 = property class="Bool (strict)"() -> ("Value"=w5437:bool)  [unwired: 2 in, 2 out]
                n2270 = property on="method" class="Ring (strict)"() -> ("Value"=w5440:i32)  [unwired: 2 in, 2 out]
                n2271 = Bundle("Value"=w5442, "Value"=w5441, "Value"=w5440, "Value"=w5439, "Value"=w5437) -> (w5438:T36)  [unwired: 1 out]
              }
              frame #1 {
                n2272 = property on="background subtraction method" class="Ring (strict)"() -> ("Value"=w5464:u16)  [unwired: 2 in, 2 out]
                n2273 = property on="special background/filter operations" class="Ring (strict)"() -> ("Value"=w5465:u16)  [unwired: 2 in, 2 out]
                n2274 = property on="subtraction type" class="Ring (strict)"() -> ("Value"=w5463:u16)  [unwired: 2 in, 2 out]
                n2275 = property on="post interp amplitude/field modifier" class="Ring (strict)"() -> ("Value"=w5462:u16)  [unwired: 2 in, 2 out]
                n2276 = property on="gamma" class="DigNum (strict)"() -> ("Value"=w5448:dbl)  [unwired: 2 in, 2 out]
                n2277 = property on="F" class="DigNum (strict)"() -> ("Value"=w5454:dbl)  [unwired: 2 in, 2 out]
                n2278 = property on="algorithm" class="Enum (strict)"() -> ("Value"=w5450:T8)  [unwired: 2 in, 2 out]
                n2279 = property on="f" class="DigNum (strict)"() -> ("Value"=w5446:dbl)  [unwired: 2 in, 2 out]
                n2280 = property on="amp" class="DigNum (strict)"() -> ("Value"=w5453:dbl)  [unwired: 2 in, 2 out]
                n2281 = property class="Bool (strict)"() -> ("Value"=w5461:bool)  [unwired: 2 in, 2 out]
                n2282 = property on="low cutoff" class="DigNum (strict)"() -> ("Value"=w5457:dbl)  [unwired: 2 in, 2 out]
                n2283 = property on="filter type" class="Enum (strict)"() -> ("Value"=w5460:T5)  [unwired: 2 in, 2 out]
                n2284 = property on="polynomial order" class="DigNum (strict)"() -> ("Value"=w5449:u8)  [unwired: 2 in, 2 out]
                n2285 = property on="amp" class="DigNum (strict)"() -> ("Value"=w5445:dbl)  [unwired: 2 in, 2 out]
                n2286 = property on="gamma" class="DigNum (strict)"() -> ("Value"=w5452:dbl)  [unwired: 2 in, 2 out]
